vi "Write.vi"(6 "Append Index":i32, 8 "error in (no error)":errorcluster, 9 "Notes":string, 10 "Data (Dictionary)":T1[](array[typedef]), 11 "Data.TDMS in":refnum<class "LV-Data.TDMS.lvclass">) -> (0 "error out":errorcluster, 3 "Data.TDMS out":refnum<class "LV-Data.TDMS.lvclass">, 5 "Path out":path)   [LabVIEW 2019, in "LV-Data.TDMS.lvclass"]
uses:
  LV-Data.TDMS.lvclass
  C:/Users/patrick/Documents/GitHub/LV-Data/src/LV-Data/LV-Data.lvclass
  LV-Data/Typedefs/Dictionary--cluster.ctl
  LV-Data.TDMS.lvclass/LV-Data.TDMS.ctl
  LV-Data/Typedefs/Operation--enum.ctl
  LV-Data/LV-Data.lvclass/LV-Data.ctl
  LV-Data/LV-Data.lvclass
  Macros/Conversion.lvclass
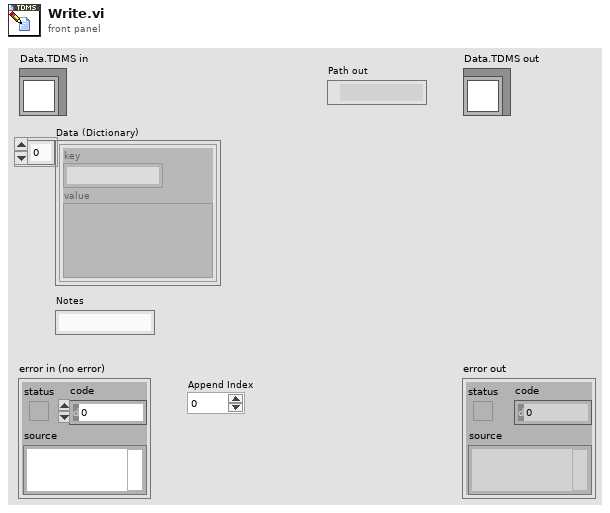
[diagram p1: front panel]
types:
  T1 = typedef "LV-Data.lvclass/Dictionary--cluster.ctl" = cluster{"key":string, "value":variant}
  T2 = typedef "LV-Data.lvclass/Operation--enum.ctl" = enum16{"Read", "Write", "Write + Append"}
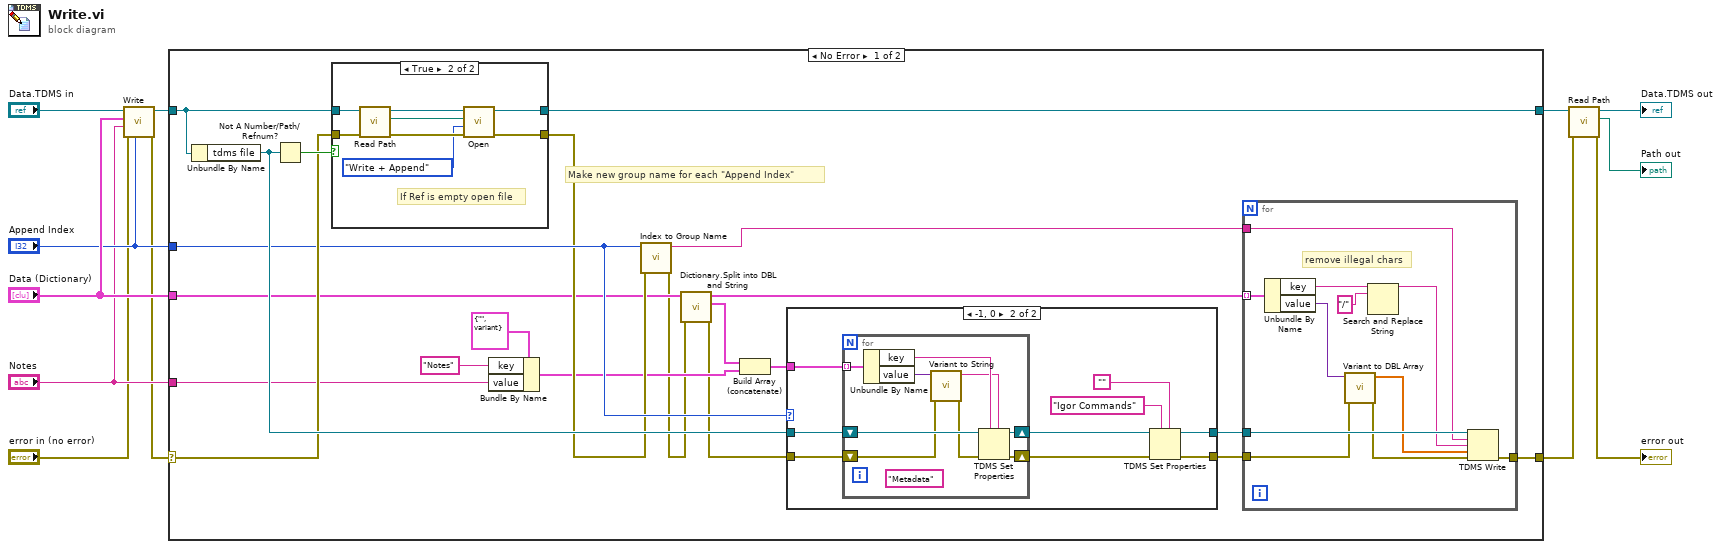
[diagram p0: block diagram]
diagram:
  n1 = call-parent "Write.vi"("Append Index"="Append Index", "error in (no error)"="error in (no error)", "Notes"="Notes", "Data (Dictionary)"="Data (Dictionary)", "Data in"="Data.TDMS in") -> ("error out"=w1:errorcluster, "Data out"=w6:refnum<class "LV-Data.TDMS.lvclass">)  [unwired: 4 in, 1 out]
  n2 = case shown="No Error" w1 {
    selector: w1 -> [w26 w76]
    tunnel: [w30 w76] -> w10
    tunnel: w6 -> [w33 w75]
    tunnel: [w29 w75] -> w12
    tunnel: "Data (Dictionary)" -> [w22 _]
    tunnel: "Notes" -> [w16 _]
    tunnel: "Append Index" -> [w25 _]
    frame No Error {
      # "Make new group name for each \"Append Index\""
      n3 = Unbundle By Name(w33) -> ("tdms file"=w27:refnum<k34>)
      n4 = Not A Number/Path/Refnum?(number/path/refnum=w27) -> (NaN/Path/Refnum?=w28:bool)
      n5 = case shown="True" w28 {
        tunnel: w33 -> [w34 w43]
        tunnel: [w34 w38] -> w29
        tunnel: [w35 w39] -> w24
        tunnel: w26 -> [w35 w40]
        frame False {
        }
        frame True {
          # "If Ref is empty open file"
          n6 = call "Read Path.vi"("error in (no error)"=w40, "Data Save"=w43) -> ("error out"=w42:errorcluster, "Path"=w37:path, "Data Save out"=w41:refnum<class "LV-Data.TDMS.lvclass">)  [unwired: 7 in]
          n7 = call-dynamic "Open.vi"("error in (no error)"=w42, "Operation"=Operation--enum."Write + Append", "Path"=w37, "Data.TDMS in"=w41) -> ("error out"=w39:errorcluster, "Data.TDMS out"=w38:refnum<class "LV-Data.TDMS.lvclass">)  [unwired: 6 in]
        }
      }
      n8 = Bundle By Name(cluster=T1 {"key"="", "value"=variant} ("input cluster"), "key"="Notes", "value"=w16) -> (w15:T1)
      n9 = call "Index to Group Name.vi"("error in (no error)"=w24, "Append Index"=w25) -> ("error out"=w14:errorcluster, "group name in (Untitled)"=w23:string)  [unwired: 8 in]
      n10 = call "Dictionary.Split into DBL and String.vi"("error in (no error)"=w14, "Data (Dictionary)"=w22) -> ("error out"=w13:errorcluster, "Data (Dictionary) (String)"=w19:T1[], "Data (Dictionary) (Dbl)"=w21:T1[])  [unwired: 7 in]
      n11 = Build Array (concatenate)(w19, w15) -> (w20:T1[])
      n12 = case shown="-1, 0" w25 {
        tunnel: w13 -> [w55 w58]
        tunnel: [w55 w63] -> w32
        tunnel: [w56 w62] -> w31
        tunnel: w27 -> [w56 w59]
        tunnel: w20 -> [_ w57]
        frame Default {
        }
        frame -1, 0 {
          n13 = for {
            shift-right: [w74] -> w65
            shift-left: w59 -> [w72]
            shift-right: [w73] -> w64
            shift-left: w58 -> [w67]
            tunnel: w57 -> [w71] mode=indexing
            (unwired) "Metadata" ("attrib name")
            n14 = Unbundle By Name(w71) -> ("key"=w70:string, "value"=w69:variant)
            n15 = call "Variant to String.vi"("error in (no error)"=w67, "Data (Variant)"=w69) -> ("error out"=w66:errorcluster, "String"=w68:string)  [unwired: 8 in]
            n16 = TDMS Set Properties(5:w68, 7:w70, 8:w66, 11:w72) -> (0:w73:errorcluster, 3:w74:refnum<k34>)  [unwired: 2 in, 2 out]
          }
          n17 = TDMS Set Properties(5:"", 7:"Igor Commands" ("attrib name"), 8:w64, 11:w65) -> (0:w63:errorcluster, 3:w62:refnum<k34>)  [unwired: 2 in, 2 out]
        }
      }
      n18 = for {
        tunnel: w21 -> [w50] mode=indexing
        tunnel: w32 -> [w48]
        tunnel: w31 -> [w53]
        tunnel: [w52] -> w30
        tunnel: w23 -> [w47]
        # "remove illegal chars"
        n19 = Unbundle By Name(w50) -> ("key"=w51:string, "value"=w46:variant)
        n20 = call "Variant to DBL Array.vi"("error in (no error)"=w48, "Data (Variant)"=w46) -> ("error out"=w49:errorcluster, "1D Array"=w44:dbl[])  [unwired: 7 in, 1 out]
        n21 = Search and Replace String(input string=w51, search string="/") -> (result string=w45:string)  [unwired: 6 in, 3 out]
        n22 = TDMS Write(0:w53, 5:w47, 7:w45, 9:w44, 11:w49) -> (15:w52:errorcluster)  [unwired: 1 in, 3 out]
      }
    }
    frame Error {
    }
  }
  n23 = call "Read Path.vi"("error in (no error)"=w10, "Data Save"=w12) -> ("error out"=→"error out":errorcluster, "Path"=→"Path out":path, "Data Save out"=→"Data.TDMS out":refnum<class "LV-Data.TDMS.lvclass">)  [unwired: 7 in]
